vi "timeout.vi"(8 "error in (no error)":errorcluster, 10 "timeout_secs":u64, 11 "obj in":refnum<class "RequestBuilder.lvclass">) -> (0 "error out":errorcluster, 2 "success":bool, 3 "obj out":refnum<class "RequestBuilder.lvclass">)   [LabVIEW 2020, in "reqwest.lvlib" / "RequestBuilder.lvclass"]
uses:
  RequestBuilder.lvclass
  RequestBuilder.lvclass/RequestBuilder.ctl
  lv_reqwest_64.so
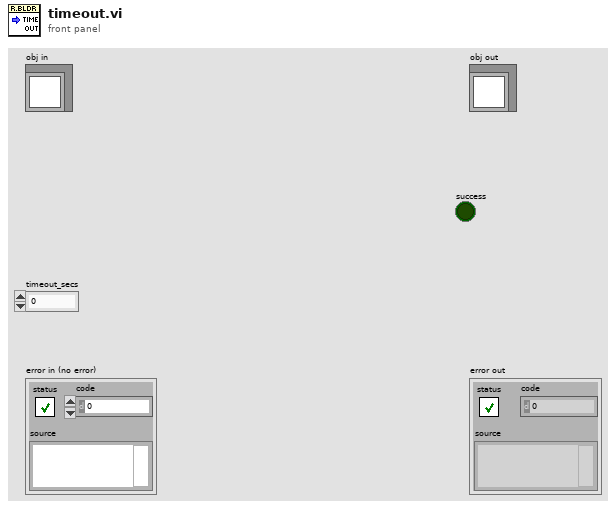
[diagram p1: front panel]
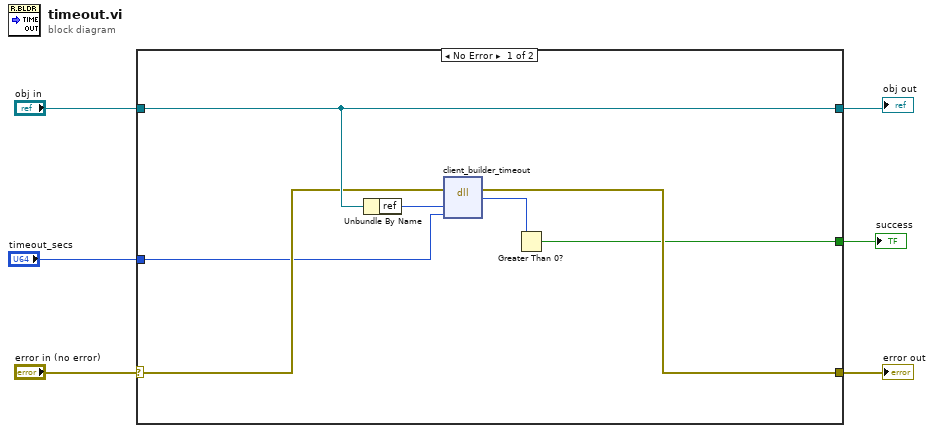
[diagram p0: block diagram]
diagram:
  n1 = case shown="No Error" "error in (no error)" {
    selector: "error in (no error)" -> [w10 w14]
    tunnel: "obj in" -> [w11 w15]
    tunnel: [w13 w14] -> w3
    tunnel: [w11 w15] -> w4
    tunnel: "timeout_secs" -> [w9 _]
    tunnel: [w7 _] -> w1
    frame No Error {
      n2 = Unbundle By Name(w11) -> ("ref"=w12:u64)
      n3 = dll-call lib="home/jim-kring/Projects/reqwest-rs-labview/lv_src/lv_reqwest_*.*" fn="client_builder_timeout"(error in=w10, "request_builder_ref"=w12, "timeout_secs"=w9) -> (error out=w13:errorcluster, "success"=w8:u8)  [unwired: 4 in, 1 out]
      n4 = Greater Than 0?(x=w8) -> (x > 0?=w7:bool)
    }
    frame Error {
    }
  }
  "error out" <- w3
  "obj out" <- w4
  "success" <- w1
